vi "Main Loop.vi"(8 "error in":errorcluster, 11 "Node in":refnum<class "BLS Chiller Template.lvclass">) -> (0 "error out":errorcluster, 3 "Node out":refnum<class "BLS Chiller Template.lvclass">)   [LabVIEW 2023, in "BLS Chiller Template.lvlib" / "BLS Chiller Template.lvclass"]
uses:
  BLS Chiller Template.lvclass
  Out Of Band/Type Defs/gRPC to Main.ctl
  Out Of Band/Type Defs/Main to gRPC.ctl
  <vilib>/ADAS Replay HIL/ADAS Plugin Utilities/AdasLvTemplate/Typedefs/Initialization States.ctl
  <vilib>/ADAS Replay HIL/ADAS Plugin Utilities/AdasLvTemplate/AdasLvTemplate.lvclass/AdasLvTemplate.ctl
  <vilib>/Platform/TimedLoop/XDataNode/timing_clust.ctl
  <vilib>/Platform/TimedLoop/XDataNode/nitl_modes.ctl
  <vilib>/Platform/TimedLoop/XDataNode/wakeup.ctl
  <vilib>/ADAS Replay HIL/ADAS Plugin Utilities/AdasLvTemplate/Typedefs/Default Plug-in States.ctl
  <vilib>/ADAS Replay HIL/ADAS Plugin Utilities/AdasLvTemplateTimeLog/Typedefs/Standard Time Events.ctl
  <vilib>/ADAS Replay HIL/ADAS Plugin Utilities/AdasLvTemplate/Typedefs/Error Options.ctl
  <vilib>/ADAS Replay HIL/Template Node/Plugin/Template Node/Template Node.lvclass/Template Node.ctl
  <vilib>/ADAS Replay HIL/ADAS Plugin Utilities/AdasLvTemplate/Time/Absolute Timed Wake.vi
  <vilib>/ADAS Replay HIL/ADAS Plugin Utilities/AdasLvTemplate/OOB Commands/OOB Comm.vi
  <vilib>/ADAS Replay HIL/ADAS Plugin Utilities/AdasLvTemplate/Time/Get Current Working Time.vi
  <vilib>/ADAS Replay HIL/ADAS Plugin Utilities/AdasLvTemplate/Time/Wake on Time.vi
  <vilib>/ADAS Replay HIL/ADAS Plugin Utilities/AdasLvTemplate/TimeLog/Write Timelog.vi
  Out Of Band/Main Loop/Main OOB Comm.vi
  Out Of Band/gRPC Loop/gRPC OOB Comm.vi
  <vilib>/ADAS Replay HIL/ADAS Plugin Utilities/AdasLvTemplate/Time/Sleep on Working Time.vi
  <vilib>/ADAS Replay HIL/ADAS Plugin Utilities/AdasLvTemplateSystemLog/Syslog Info.vi
  <vilib>/ADAS Replay HIL/ADAS Plugin Utilities/AdasLvTemplate/OOB Commands/Parse Timing Data.vi
  <vilib>/ADAS Replay HIL/ADAS Plugin Utilities/AdasLvTemplate/OOB Commands/Typecast Command ID.vi
  <vilib>/ADAS Replay HIL/ADAS Plugin Utilities/AdasLvTemplate/OOB Responses/Write Status.vi
  <vilib>/ADAS Replay HIL/ADAS Plugin Utilities/AdasLvTemplateOutOfBand/Read OOB no_mem.vi
  <vilib>/ADAS Replay HIL/ADAS Plugin Utilities/AdasLvTemplateCommon/Time/Calculate Cycle Timing Statistics.vi
  <vilib>/ADAS Replay HIL/ADAS Plugin Utilities/AdasLvTemplateCommon/Time/Calculate Delta Timing Statistics.vi
  <vilib>/ADAS Replay HIL/ADAS Plugin Utilities/AdasLvTemplate/OOB Responses/Update StatusPub Timing Stats.vi
  <vilib>/ADAS Replay HIL/ADAS Plugin Utilities/AdasLvTemplate/TimeLog/Write All States Timelog.vi
  <vilib>/ADAS Replay HIL/ADAS Plugin Utilities/AdasLvTemplate/TimeLog/Update Data Output Timing Stats.vi
  <vilib>/ADAS Replay HIL/ADAS Plugin Utilities/AdasLvTemplateSystemLog/Write to ADAS Log.vi
  <vilib>/ADAS Replay HIL/ADAS Plugin Utilities/AdasLvTemplateCommon/Byte Pack/Unpack Data.vi
  <vilib>/ADAS Replay HIL/ADAS Plugin Utilities/AdasLvTemplateCommon/Byte Pack/Unpack U64.vi
  <vilib>/ADAS Replay HIL/ADAS Plugin Utilities/AdasLvTemplateCommon/Byte Pack/Unpack Dbl.vi
  <vilib>/ADAS Replay HIL/ADAS Plugin Utilities/AdasLvTemplate/OOB Commands/Typecast Command ID.vi/33a1a329-153d-46bf-b82a-13d67c924fdc.vi
  <vilib>/ADAS Replay HIL/ADAS Plugin Utilities/AdasLvTemplate/OOB Commands/Typecast Command ID.vi/47c6e19f-85af-4ecd-9b35-4c0af7f9c4eb.vi
  <vilib>/ADAS Replay HIL/ADAS Plugin Utilities/AdasLvTemplate/OOB Responses/Send Status.vi
  <vilib>/ADAS Replay HIL/ADAS Plugin Utilities/AdasLvTemplateCommon/Byte Pack/Unpack U8.vi
  <vilib>/ADAS Replay HIL/ADAS Plugin Utilities/AdasLvTemplateTimeLog/Write All State Timelog.vi
  <vilib>/ADAS Replay HIL/ADAS Plugin Utilities/AdasLvTemplate/TimeLog/Write All Data Outputs Timelog.vi
  <vilib>/ADAS Replay HIL/ADAS Plugin Utilities/AdasLvTemplateSystemLog/Log to OS.vi
  <vilib>/ADAS Replay HIL/ADAS Plugin Utilities/AdasLvTemplateCommon/Byte Pack/Unpack U64.vi/6cead1c8-1490-489b-94c0-a6f77a877bd8.vi
  <vilib>/ADAS Replay HIL/ADAS Plugin Utilities/AdasLvTemplateCommon/Byte Pack/Unpack Dbl.vi/1ddba392-4989-4550-9efa-bf0f5b4d8642.vi
  <vilib>/ADAS Replay HIL/ADAS Plugin Utilities/AdasLvTemplate/OOB Commands/Typecast Command ID.vi/33a1a329-153d-46bf-b82a-13d67c924fdc.vi/c28b0ead-42ad-4072-80a2-aca7f2bd7ce3.vi
  <vilib>/ADAS Replay HIL/ADAS Plugin Utilities/AdasLvTemplate/OOB Commands/Typecast Command ID.vi/47c6e19f-85af-4ecd-9b35-4c0af7f9c4eb.vi/c28b0ead-42ad-4072-80a2-aca7f2bd7ce3.vi
  <vilib>/ADAS Replay HIL/ADAS Plugin Utilities/AdasLvTemplate/OOB Responses/Pack Status.vi
  <vilib>/ADAS Replay HIL/ADAS Plugin Utilities/AdasLvTemplateOutOfBand/Write OOB no_mem.vi
  <vilib>/ADAS Replay HIL/ADAS Plugin Utilities/AdasLvTemplateCommon/Byte Pack/Unpack U8.vi/dab2b46f-2b54-43c4-abff-a01388689065.vi
  <vilib>/ADAS Replay HIL/ADAS Plugin Utilities/AdasLvTemplateTimeLog/Write Standard Timelog.vi
  <vilib>/ADAS Replay HIL/ADAS Plugin Utilities/AdasLvTemplateTimeLog/Write Data Channel Timelog.vi
  <vilib>/ADAS Replay HIL/ADAS Plugin Utilities/AdasLvTemplateCommon/Byte Pack/Unpack U64.vi/6cead1c8-1490-489b-94c0-a6f77a877bd8.vi/c28b0ead-42ad-4072-80a2-aca7f2bd7ce3.vi
  <vilib>/ADAS Replay HIL/ADAS Plugin Utilities/AdasLvTemplateCommon/Byte Pack/Unpack Dbl.vi/1ddba392-4989-4550-9efa-bf0f5b4d8642.vi/c28b0ead-42ad-4072-80a2-aca7f2bd7ce3.vi
  <vilib>/ADAS Replay HIL/ADAS Plugin Utilities/AdasLvTemplate/OOB Responses/Pack Status.vi/b11e0591-7eee-4cf7-b3b4-c7ab44274ca8.vi
  <vilib>/ADAS Replay HIL/ADAS Plugin Utilities/AdasLvTemplateCommon/Byte Pack/Pack Data.vi
  <vilib>/ADAS Replay HIL/ADAS Plugin Utilities/AdasLvTemplateCommon/Byte Pack/Pack U8.vi
  <vilib>/ADAS Replay HIL/ADAS Plugin Utilities/AdasLvTemplateCommon/Byte Pack/Unpack U8.vi/dab2b46f-2b54-43c4-abff-a01388689065.vi/c28b0ead-42ad-4072-80a2-aca7f2bd7ce3.vi
  <vilib>/ADAS Replay HIL/ADAS Plugin Utilities/AdasLvTemplateTimeLog/Write Standard Timelog.vi/f085caac-7a92-4bf8-966d-28d65be49b40.vi
  <vilib>/ADAS Replay HIL/ADAS Plugin Utilities/AdasLvTemplate/Time/Get Current System Time.vi
  <vilib>/ADAS Replay HIL/ADAS Plugin Utilities/AdasLvTemplateSystemLog/Syslog to bytes.vi
  <vilib>/ADAS Replay HIL/ADAS Plugin Utilities/AdasLvTemplate/OOB Responses/Pack Status.vi/b11e0591-7eee-4cf7-b3b4-c7ab44274ca8.vi/c28b0ead-42ad-4072-80a2-aca7f2bd7ce3.vi
  <vilib>/ADAS Replay HIL/ADAS Plugin Utilities/AdasLvTemplateCommon/Byte Pack/Pack U8.vi/d26b960e-7005-4648-98c8-b1ee87e9a649.vi
  <vilib>/libnicipc/SubVIs/check_error.vi
  <vilib>/libnicipc/Get Element Write Position.vi
  <vilib>/ADAS Replay HIL/ADAS Plugin Utilities/AdasLvTemplateCommon/Byte Pack/Pack U16.vi
  <vilib>/ADAS Replay HIL/ADAS Plugin Utilities/AdasLvTemplateCommon/Byte Pack/Pack U64.vi
  <vilib>/ADAS Replay HIL/ADAS Plugin Utilities/AdasLvTemplateCommon/Byte Pack/Pack U8.vi/d26b960e-7005-4648-98c8-b1ee87e9a649.vi/c28b0ead-42ad-4072-80a2-aca7f2bd7ce3.vi
  <vilib>/ADAS Replay HIL/ADAS Plugin Utilities/AdasLvTemplateCommon/Byte Pack/Pack U16.vi/b7087905-2eb2-4c97-90c8-7b5681595cff.vi
  <vilib>/ADAS Replay HIL/ADAS Plugin Utilities/AdasLvTemplateCommon/Byte Pack/Pack U64.vi/5a0cf944-c84d-49bc-a60a-1e686f5e9f60.vi
  <vilib>/ADAS Replay HIL/ADAS Plugin Utilities/AdasLvTemplateCommon/Byte Pack/Pack U16.vi/b7087905-2eb2-4c97-90c8-7b5681595cff.vi/c28b0ead-42ad-4072-80a2-aca7f2bd7ce3.vi
  <vilib>/ADAS Replay HIL/ADAS Plugin Utilities/AdasLvTemplateCommon/Byte Pack/Pack U64.vi/5a0cf944-c84d-49bc-a60a-1e686f5e9f60.vi/c28b0ead-42ad-4072-80a2-aca7f2bd7ce3.vi
  Out Of Band/gRPC Loop/Class to gRPC_to_Main.vi
  Out Of Band/Main Loop/Class to Main_to_gRPC.vi
  <vilib>/ADAS Replay HIL/ADAS Plugin Utilities/AdasLvTemplate/OOB Commands/Parse Start Restart Data.vi
  <vilib>/ADAS Replay HIL/ADAS Plugin Utilities/AdasLvTemplate/OOB Commands/Parse Priority Data.vi
  <vilib>/ADAS Replay HIL/AdasHilServices/Get Time.vi
  <vilib>/ADAS Replay HIL/AdasHilServices/nS Sleep.vi
  <vilib>/Utility/error.llb/Error Cluster From Error Code.vi
  <vilib>/ADAS Replay HIL/AdasHilServices/Wake On Time Advanced.vi
  <vilib>/libnicipc/SubVIs/Get Element Info Variant.vi
  <vilib>/libnicipc/Notify Of New Write.vi
  <vilib>/ADAS Replay HIL/ADAS Plugin Utilities/AdasLvTemplate/AdasLvTemplate.lvclass
  <vilib>/Platform/TimedLoop/XDataNode/XDataNode.xnode
  BLS Chiller Template.lvclass/BLS Chiller Template.ctl
  <vilib>/ADAS Replay HIL/Template Node/Plugin/Template Node/Template Node.lvclass
  <vilib>/ADAS Replay HIL/ADAS Plugin Utilities/AdasLvTemplateTimeLog/AdasLvTemplateTimeLog.lvlib
  <vilib>/Platform/TimedLoop/XDataNode/XDNodeRunTimeDep.lvlib
panel:
  out "Main to gRPC":T1
  out "gRPC to Main":T2
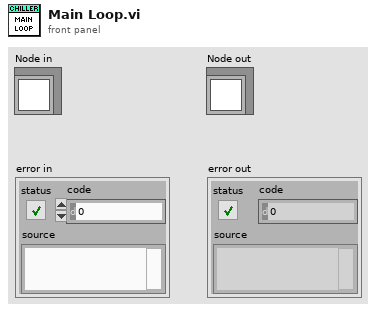
[diagram p1: front panel]
types:
  T1 = typedef "BLS Chiller Template.lvlib/BLS Chiller Template.lvclass/Main to gRPC.ctl" = cluster{"void":bool}
  T2 = typedef "BLS Chiller Template.lvlib/BLS Chiller Template.lvclass/gRPC to Main.ctl" = cluster{"void":bool}
  T3 = typedef "AdasLvTemplate.lvlib/AdasLvTemplate.lvclass/Initialization States.ctl" = enum16{"Entry Init", "Ready", "Exit Init", "Error"}
  T4 = typedef "AdasLvTemplate.lvlib/AdasLvTemplate.lvclass/Default Plug-in States.ctl" = enum16{"Start", "Pause", "Restart", "Execute Logic", "Housekeeping", "Error", "Shutdown"}
  T5 = typedef "AdasLvTemplateTimeLog.lvlib/Standard Time Events.ctl" = enum16{"Start Sleep", "Wakeup", "End of Execution", "Start of Housekeeping", "Target Wake Time", "Channel T0", "Channel TX_in", "Channel RX", "Channel out", "Target Channel out "}
  T6 = typedef "AdasLvTemplate.lvlib/AdasLvTemplate.lvclass/Error Options.ctl" = enum16{"Clear and Log Only", "Pause on Error", "Restart on Error", "Pause on Warning", "Restart on Warning"}
  T7 = typedef "XDNodeRunTimeDep.lvlib/timing_clust.ctl" = cluster{"Expected End [f-1]":u64, "Actual End [f-1]":u64, "Finished Late? [f-1]":bool, "Expected End [i-1]":u64, "Actual End [i-1]":u64, "Finished Late? [i-1]":bool, "Expected Start [i]":u64, "Actual Start [i]":u64, "Expected Start [f]":u64, "Actual Start [f]":u64, "Source Name":string, "Structure Name":string, "Period":i64, "Deadline":i64, "Offset":i64, "Start":i64, "Priority":i32, "Timeout":i32, "Mode":T8, "Wakeup Reason":T9, "Error":errorcluster, "Source Type":string, "Secondary Source Type":string, "Global End Time":u64, "Global Start Time":u64, "Frame Duration":u64, "Iteration Duration":u64, "Assigned CPU":i32, "I/O Scan Engine Mode":u32}
  T8 = typedef "XDNodeRunTimeDep.lvlib/nitl_modes.ctl" = enum32{"No Change", "Process missed periods, maintain original phase", "Discard missed periods, maintain original phase", "Process missed periods, ignore original phase", "Discard missed periods, ignore original phase"}
  T9 = typedef "XDNodeRunTimeDep.lvlib/wakeup.ctl" = enum32{"Normal", "Aborted", "Asynchronous wakeup", "Timing source error", "Timed loop error", "Timeout"}
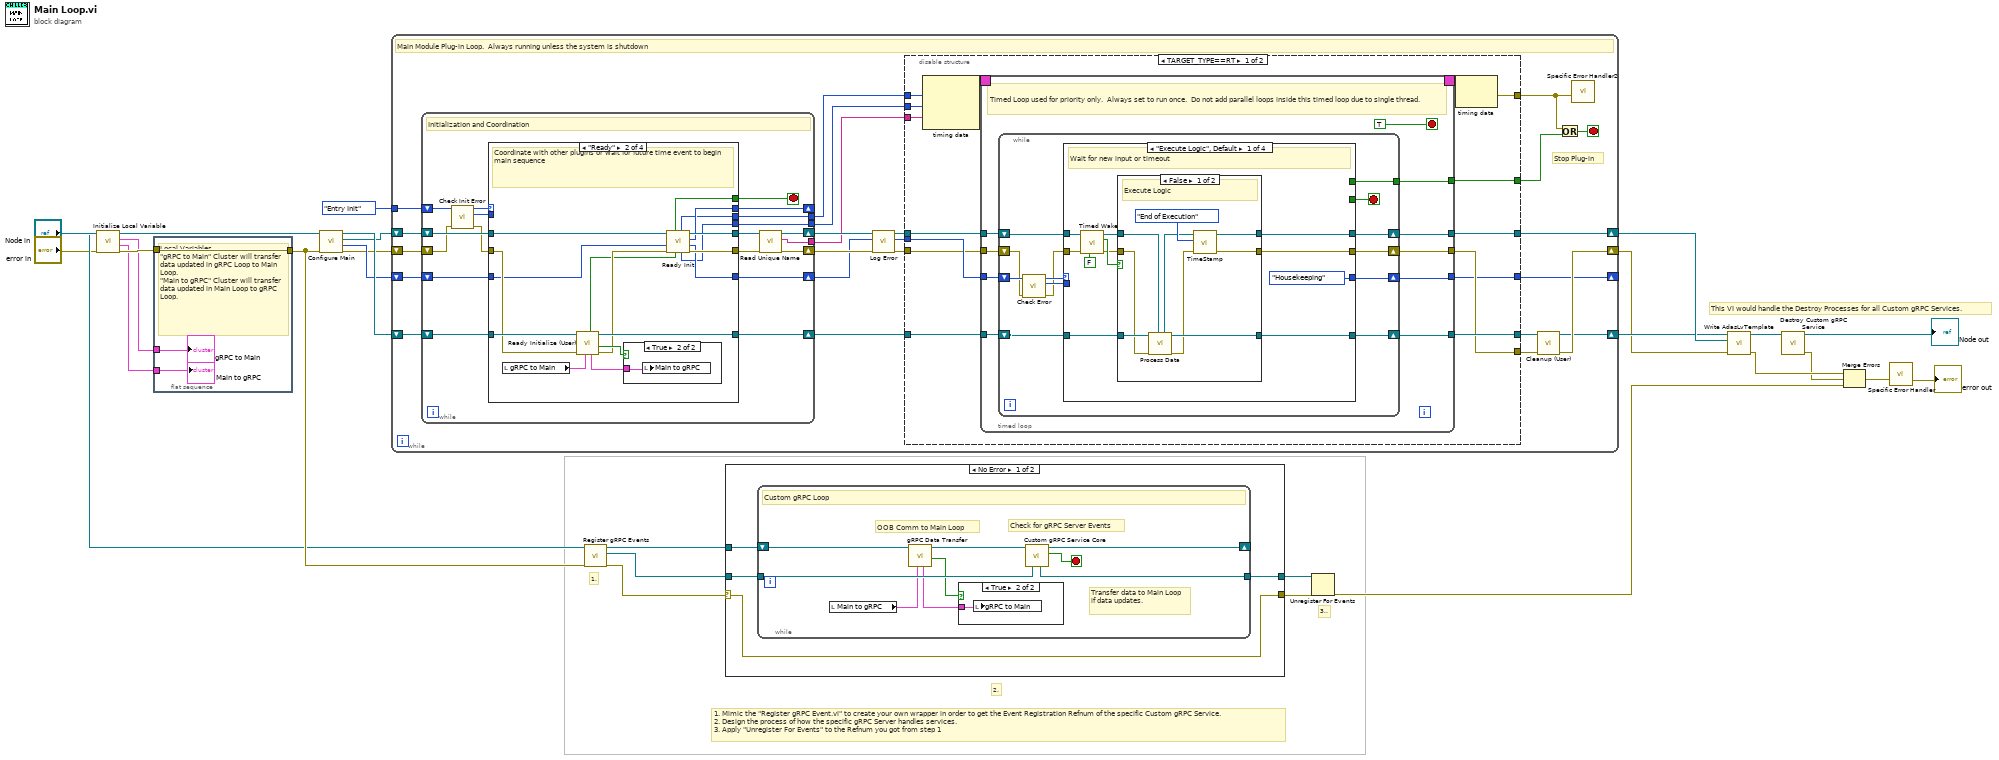
[diagram p0: block diagram]
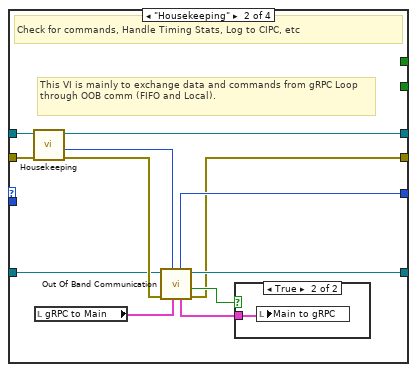
[diagram p5: hidden frame]
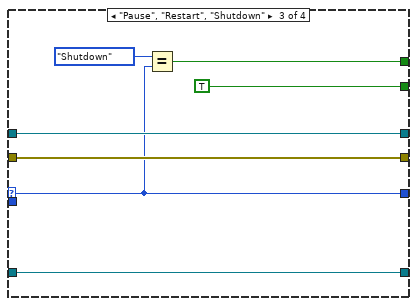
[diagram p7: hidden frame]
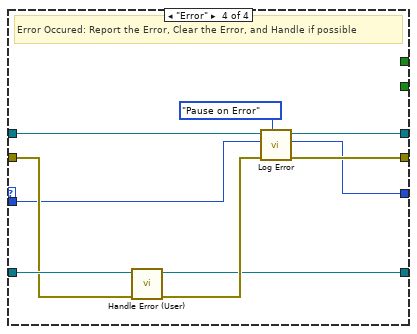
[diagram p8: hidden frame]
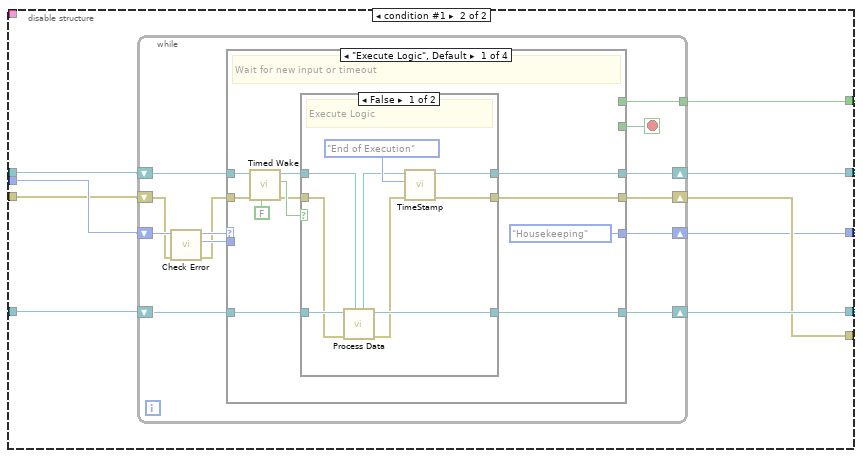
[diagram p9: hidden frame]
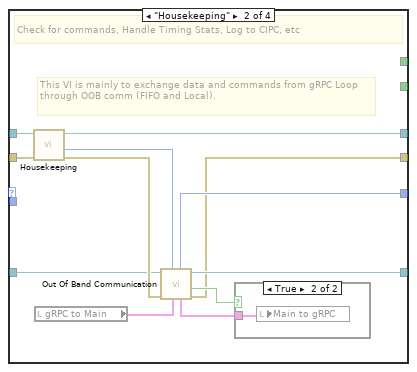
[diagram p11: hidden frame]
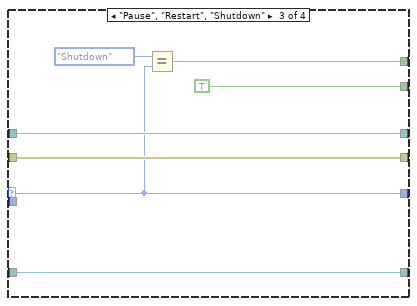
[diagram p13: hidden frame]
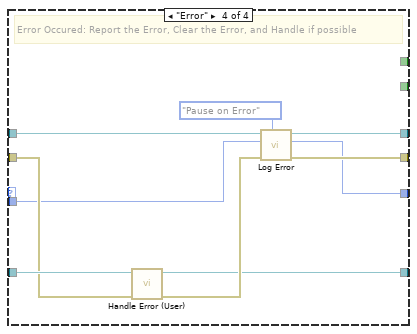
[diagram p14: hidden frame]
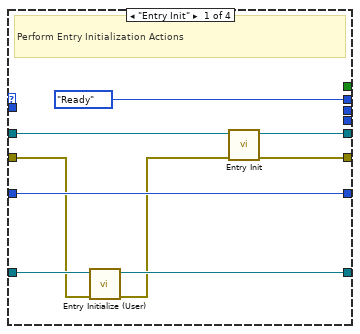
[diagram p15: hidden frame]
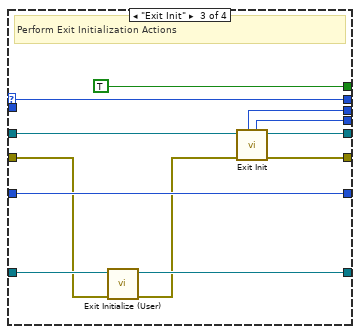
[diagram p17: hidden frame]
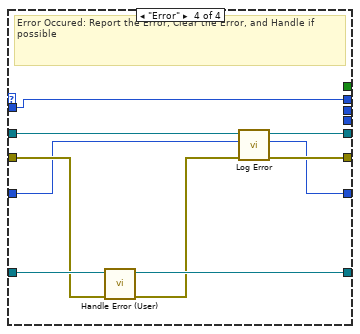
[diagram p18: hidden frame]
diagram:
  # "This VI would handle the Destroy Processes for all Custom gRPC Services."
  # "3.."
  # "2."
  # "1."
  # "1. Mimic the \"Register gRPC Event.vi\" to create your own wrapper in order to get the Event Registration Refnum of the specific Custom gRPC Service.\n2. Design the process of how the specific gRPC Server handles services.\n3. Apply \"Unregister For Events\" to the Refnum you got from step 1"
  n1 = call "Initialize Local Variable.vi"("error in"="error in", "Timed Node in"="Node in") -> ("error out"=w5:errorcluster, "Main to gRPC"=w3:T1, "gRPC to Main"=w4:T2, "Timed Node out"=w7:refnum<class "BLS Chiller Template.lvclass">)  [unwired: 6 in]
  n2 = flat-sequence {
    tunnel: w5 -> [w30]
    tunnel: [w30] -> w9
    tunnel: w4 -> [w29]
    tunnel: w3 -> [w28]
    frame #0 {
      # "Local Variables \n\"gRPC to Main\" Cluster will transfer data updated in gRPC Loop to Main Loop.\n\"Main to gRPC\" Cluster will transfer data updated in Main Loop to gRPC Loop."
      "gRPC to Main" <- w29
      "Main to gRPC" <- w28
    }
  }
  n3 = call <vilib>:"Configure Main.vi"("error in (no error)"=w9, "Template Node in"=w7) -> ("error out"=w21:errorcluster, "Initial State"=w22:T4, "AdasLvTemplate"=w20:refnum<class "AdasLvTemplate.lvclass">, "Template Node out"=w23:refnum<class "BLS Chiller Template.lvclass">)  [unwired: 6 in]
  n4 = while {
    shift-right: [w38] -> w27
    shift-left: w20 -> [w51]
    shift-right: [w36] -> _
    shift-left: w22 -> [w53]
    shift-right: [w46] -> w26
    shift-left: w23 -> [w54]
    shift-right: [w47] -> w25
    shift-left: w21 -> [w52]
    tunnel: Initialization_States."Entry Init" -> [w50]
    stop <- w45 stop-if-true
    # "Stop Plug-in"
    # "Main Module Plug-in Loop.  Always running unless the system is shutdown"
    n5 = while {
      shift-right: [w248] -> _
      shift-left: w50 -> [w242]
      shift-right: [w231] -> w49
      shift-left: w51 -> [w246]
      shift-right: [w233] -> w48
      shift-left: w52 -> [w240]
      shift-right: [w243] -> w43
      shift-left: w54 -> [w244]
      shift-right: [w237] -> w44
      shift-left: w53 -> [w236]
      tunnel: [w235] -> w31
      tunnel: [w234] -> w32
      tunnel: [w230] -> w33
      stop <- w247 stop-if-true
      # "Initialization and Coordination"
      n6 = call <vilib>:"Check Init Error.vi"("error in"=w240, "State"=w242) -> ("error out"=w239:errorcluster, "Next State"=w238:T3, "State"=w241:T3)  [unwired: 7 in]
      n7 = case shown="\"Ready\"" w241 {
        selector: w241 -> [_ _ w287 _]
        tunnel: [Initialization_States."Ready" w264 w287 w295] -> w248
        tunnel: [_ w259 TRUE ("stop 2") _] -> w247
        tunnel: w246 -> [w250 w274 w276 w290]
        tunnel: [w255 w273 w283 w297] -> w232
        tunnel: [w249 w267 w282 w296] -> w245
        tunnel: w238 -> [_ _ _ w295]
        tunnel: w239 -> [w251 w265 w277 w291]
        tunnel: w244 -> [w254 w272 w280 w294]
        tunnel: [w253 w271 w279 w293] -> w243
        tunnel: [w256 w262 w281 w289] -> w237
        tunnel: w236 -> [w256 w261 w281 w288]
        tunnel: [_ w263 w285 _] -> w235
        tunnel: [_ w260 w284 _] -> w234
        frame "Entry Init" {
          # "Perform Entry Initialization Actions"
          n8 = call "Entry Initialize (User).vi"("error in"=w251, "Node in"=w254) -> ("error out"=w252:errorcluster, "Node out"=w253:refnum<class "BLS Chiller Template.lvclass">)  [unwired: 8 in]
          n9 = call <vilib>:"Entry Init.vi"("error in (no error)"=w252, "AdasLvTemplate in"=w250) -> ("error out"=w249:errorcluster, "AdasLvTemplate out"=w255:refnum<class "AdasLvTemplate.lvclass">)  [unwired: 8 in]
        }
        frame "Ready" {
          # "Coordinate with other plugins or wait for future time event to begin main sequence"
          n10 = local read "gRPC to Main"() -> (w269:T2)
          n11 = call "Ready Initialize (User).vi"("gRPC to Main"=w269, "error in (no error)"=w265, "Node in"=w272) -> ("error out"=w266:errorcluster, "Update Local Variable"=w270:bool, "Node out"=w271:refnum<class "BLS Chiller Template.lvclass">, "Main to gRPC"=w268:T1, "User Ready Init Done"=w258:bool)  [unwired: 4 in]
          n12 = case shown="True" w270 {
            tunnel: w268 -> [_ w275]
            frame False {
            }
            frame True {
              n13 = local write "Main to gRPC"(w275) -> ()
            }
          }
          n14 = call <vilib>:"Ready Init.vi"("User Ready Init Done"=w258, "error in (no error)"=w266, "Plug-in State in"=w261, "AdasLvTemplate in"=w274) -> ("error out"=w267:errorcluster, "Plug-in State"=w262:T4, "Initialization State"=w264:T3, "AdasLvTemplate out"=w273:refnum<class "AdasLvTemplate.lvclass">, "Processor"=w260:i32, "Priority"=w263:i32, "Shutdown?"=w259:bool)  [unwired: 1 in]
        }
        frame "Exit Init" {
          # "Perform Exit Initialization Actions"
          n15 = call "Exit Initialize (User).vi"("error in"=w277, "Node in"=w280) -> ("error out"=w278:errorcluster, "Node out"=w279:refnum<class "BLS Chiller Template.lvclass">)  [unwired: 8 in]
          n16 = call <vilib>:"Exit Init.vi"("error in (no error)"=w278, "AdasLvTemplate in"=w276) -> ("error out"=w282:errorcluster, "AdasLvTemplate out"=w283:refnum<class "AdasLvTemplate.lvclass">, "Processor"=w284:i32, "Priority"=w285:i32)  [unwired: 5 in, 1 out]
        }
        frame "Error" {
          # "Error Occured: Report the Error, Clear the Error, and Handle if possible"
          n17 = call "Handle Error (User).vi"("error in"=w291, "Node in"=w294) -> ("error out"=w292:errorcluster, "Node out"=w293:refnum<class "BLS Chiller Template.lvclass">)  [unwired: 8 in]
          n18 = call <vilib>:"Log Error.vi"("error in (no error)"=w292, "Plug-in State in"=w288, "AdasLvTemplate in"=w290) -> ("error out"=w296:errorcluster, "Plug-in State out"=w289:T4, "AdasLvTemplate out"=w297:refnum<class "AdasLvTemplate.lvclass">)  [unwired: 6 in]
        }
      }
      n19 = call <vilib>:"Read Unique Name.vi"("error in"=w245, "AdasLvTemplate in"=w232) -> ("error out"=w233:errorcluster, "Unique Name"=w230:string, "AdasLvTemplate out"=w231:refnum<class "AdasLvTemplate.lvclass">)  [unwired: 7 in]
    }
    n20 = call <vilib>:"Log Error.vi"("error in (no error)"=w48, "Plug-in State in"=w44, "AdasLvTemplate in"=w49) -> ("error out"=w40:errorcluster, "Plug-in State out"=w41:T4, "AdasLvTemplate out"=w39:refnum<class "AdasLvTemplate.lvclass">)  [unwired: 6 in]
    n21 = disable-structure shown="TARGET_TYPE==RT" {
      disable-tunnel: w43 -> [w67 w163]
      disable-tunnel: [w66 w162] -> w42
      disable-tunnel: w41 -> [w65 w161]
      disable-tunnel: w40 -> [w64 w160]
      disable-tunnel: w39 -> [w63 w159]
      disable-tunnel: [w62 w158] -> w38
      disable-tunnel: [w61 w157] -> w37
      disable-tunnel: [w60 w156] -> w36
      disable-tunnel: [w59 w155] -> w35
      disable-tunnel: [w58 _] -> w34
      disable-tunnel: w33 -> [w57 _]
      disable-tunnel: w32 -> [w56 _]
      disable-tunnel: w31 -> [w55 _]
      frame condition #0 (active) {
        n22 = node-c288(w55, w56, w57) -> (w69:T7)
        n23 = timed-loop {
          timing: w69 -> [_]
          timing-out: [_] -> w68
          tunnel: w67 -> [w79]
          tunnel: [w78] -> w66
          tunnel: w65 -> [w77]
          tunnel: w64 -> [w76]
          tunnel: w63 -> [w75]
          tunnel: [w74] -> w62
          tunnel: [w73] -> w61
          tunnel: [w72] -> w60
          tunnel: [w71] -> w59
          stop <- TRUE stop-if-true
          # "Timed Loop used for priority only.  Always set to run once.  Do not add parallel loops inside this timed loop due to single thread."
          n24 = while {
            shift-right: [w92] -> w72
            shift-left: w77 -> [w86]
            tunnel: [w90] -> w71
            shift-right: [w88] -> w74
            shift-left: w75 -> [w89]
            shift-right: [w87] -> w73
            shift-left: w76 -> [w83]
            shift-right: [w81] -> w78
            shift-left: w79 -> [w82]
            stop <- w91 stop-if-true
            n25 = call <vilib>:"Check Error.vi"("error in"=w83, "State"=w86) -> ("error out"=w80:errorcluster, "Next State"=w84:T4, "State"=w85:T4)  [unwired: 7 in]
            n26 = case shown="\"Execute Logic\", Default" w85 {
              selector: w85 -> [_ _ w130 _]
              tunnel: [Default_Plug-in_States."Housekeeping" ("Default Plug-in States") w123 w130 w138] -> w92
              tunnel: [_ _ TRUE ("stop 2") _] -> w91
              tunnel: [_ _ w129 _] -> w90
              tunnel: w89 -> [w97 w127 w135 w139]
              tunnel: [w99 w125 w135 w145] -> w88
              tunnel: [w93 w116 w133 w144] -> w87
              tunnel: w84 -> [_ _ _ w136]
              tunnel: w80 -> [w98 w126 w133 w142]
              tunnel: w82 -> [w96 w121 w132 w143]
              tunnel: [w95 w120 w132 w140] -> w81
              frame "Execute Logic", Default {
                # "Wait for new input or timeout"
                n27 = call <vilib>:"Timed Wake.vi"("Data Driven Timing"=FALSE, "error in (no error)"=w98, "AdasLvTemplate in"=w97) -> ("error out"=w100:errorcluster, "Timeout"=w103:bool, "AdasLvTemplate out"=w101:refnum<class "AdasLvTemplate.lvclass">)  [unwired: 4 in, 2 out]
                n28 = case shown="False" w103 {
                  tunnel: [w108 w115] -> w99
                  tunnel: w101 -> [w106 w115]
                  tunnel: [w104 w114] -> w93
                  tunnel: w100 -> [w109 w114]
                  tunnel: w96 -> [w111 w113]
                  tunnel: [w110 w113] -> w95
                  frame False {
                    # "Execute Logic"
                    n29 = call "Process Data.vi"("AdasLvTemplate in"=w106, "error in"=w109, "Node in"=w111) -> ("error out"=w107:errorcluster, "Node out"=w110:refnum<class "BLS Chiller Template.lvclass">, "AdasLvTemplate out"=w105:refnum<class "AdasLvTemplate.lvclass">)  [unwired: 6 in]
                    n30 = call <vilib>:"TimeStamp.vi"("error in (no error)"=w107, "Event"=Standard_Time_Events."End of Execution", "AdasLvTemplate in"=w105) -> ("error out"=w104:errorcluster, "AdasLvTemplate out"=w108:refnum<class "AdasLvTemplate.lvclass">)  [unwired: 7 in]
                  }
                  frame True {
                    # "Timeout"
                  }
                }
              }
              frame "Housekeeping" {
                # "This VI is mainly to exchange data and commands from gRPC Loop through OOB comm (FIFO and Local)."
                # "Check for commands, Handle Timing Stats, Log to CIPC, etc"
                n31 = call <vilib>:"Housekeeping.vi"("error in (no error)"=w126, "AdasLvTemplate in"=w127) -> ("error out"=w122:errorcluster, "State"=w124:T4, "AdasLvTemplate out"=w125:refnum<class "AdasLvTemplate.lvclass">)  [unwired: 7 in]
                n32 = local read "gRPC to Main"() -> (w119:T2)
                n33 = call "Out Of Band Communication.vi"("gRPC to Main"=w119, "State In"=w124, "error in"=w122, "Node in"=w121) -> ("error out"=w116:errorcluster, "Update Local Variable"=w117:bool, "Node out"=w120:refnum<class "BLS Chiller Template.lvclass">, "Main to gRPC"=w118:T1, "State Out"=w123:T4)  [unwired: 3 in]
                n34 = case shown="True" w117 {
                  tunnel: w118 -> [_ w128]
                  frame False {
                  }
                  frame True {
                    n35 = local write "Main to gRPC"(w128) -> ()
                  }
                }
              }
              frame "Pause", "Restart", "Shutdown" {
                n36 = Equal?(x=Default_Plug-in_States."Shutdown" ("Default Plug-in States"), y=w130) -> (x = y?=w129:bool)
              }
              frame "Error" {
                # "Error Occured: Report the Error, Clear the Error, and Handle if possible"
                n37 = call "Handle Error (User).vi"("error in"=w142, "Node in"=w143) -> ("error out"=w141:errorcluster, "Node out"=w140:refnum<class "BLS Chiller Template.lvclass">)  [unwired: 8 in]
                n38 = call <vilib>:"Log Error.vi"("Action"=Error_Options."Pause on Error", "error in (no error)"=w141, "Plug-in State in"=w136, "AdasLvTemplate in"=w139) -> ("error out"=w144:errorcluster, "Plug-in State out"=w138:T4, "AdasLvTemplate out"=w145:refnum<class "AdasLvTemplate.lvclass">)  [unwired: 5 in]
              }
            }
          }
        }
        n39 = node-c288(w68) -> (w58:errorcluster)
      }
      frame condition #1 {
        n40 = while {
          shift-right: [w176] -> w156
          shift-left: w161 -> [w170]
          tunnel: [w174] -> w155
          shift-right: [w172] -> w158
          shift-left: w159 -> [w173]
          shift-right: [w171] -> w157
          shift-left: w160 -> [w167]
          shift-right: [w165] -> w162
          shift-left: w163 -> [w166]
          stop <- w175 stop-if-true
          n41 = call <vilib>:"Check Error.vi"("error in"=w167, "State"=w170) -> ("error out"=w164:errorcluster, "Next State"=w168:T4, "State"=w169:T4)  [unwired: 7 in]
          n42 = case shown="\"Execute Logic\", Default" w169 {
            selector: w169 -> [_ _ w214 _]
            tunnel: [Default_Plug-in_States."Housekeeping" ("Default Plug-in States") w207 w214 w222] -> w176
            tunnel: [_ _ TRUE ("stop 2") _] -> w175
            tunnel: [_ _ w213 _] -> w174
            tunnel: w173 -> [w181 w211 w219 w223]
            tunnel: [w183 w209 w219 w229] -> w172
            tunnel: [w177 w200 w217 w228] -> w171
            tunnel: w168 -> [_ _ _ w220]
            tunnel: w164 -> [w182 w210 w217 w226]
            tunnel: w166 -> [w180 w205 w216 w227]
            tunnel: [w179 w204 w216 w224] -> w165
            frame "Execute Logic", Default {
              # "Wait for new input or timeout"
              n43 = call <vilib>:"Timed Wake.vi"("Data Driven Timing"=FALSE, "error in (no error)"=w182, "AdasLvTemplate in"=w181) -> ("error out"=w184:errorcluster, "Timeout"=w187:bool, "AdasLvTemplate out"=w185:refnum<class "AdasLvTemplate.lvclass">)  [unwired: 4 in, 2 out]
              n44 = case shown="False" w187 {
                tunnel: [w192 w199] -> w183
                tunnel: w185 -> [w190 w199]
                tunnel: [w188 w198] -> w177
                tunnel: w184 -> [w193 w198]
                tunnel: w180 -> [w195 w197]
                tunnel: [w194 w197] -> w179
                frame False {
                  # "Execute Logic"
                  n45 = call "Process Data.vi"("AdasLvTemplate in"=w190, "error in"=w193, "Node in"=w195) -> ("error out"=w191:errorcluster, "Node out"=w194:refnum<class "BLS Chiller Template.lvclass">, "AdasLvTemplate out"=w189:refnum<class "AdasLvTemplate.lvclass">)  [unwired: 6 in]
                  n46 = call <vilib>:"TimeStamp.vi"("error in (no error)"=w191, "Event"=Standard_Time_Events."End of Execution", "AdasLvTemplate in"=w189) -> ("error out"=w188:errorcluster, "AdasLvTemplate out"=w192:refnum<class "AdasLvTemplate.lvclass">)  [unwired: 7 in]
                }
                frame True {
                  # "Timeout"
                }
              }
            }
            frame "Housekeeping" {
              # "This VI is mainly to exchange data and commands from gRPC Loop through OOB comm (FIFO and Local)."
              # "Check for commands, Handle Timing Stats, Log to CIPC, etc"
              n47 = call <vilib>:"Housekeeping.vi"("error in (no error)"=w210, "AdasLvTemplate in"=w211) -> ("error out"=w206:errorcluster, "State"=w208:T4, "AdasLvTemplate out"=w209:refnum<class "AdasLvTemplate.lvclass">)  [unwired: 7 in]
              n48 = local read "gRPC to Main"() -> (w203:T2)
              n49 = call "Out Of Band Communication.vi"("gRPC to Main"=w203, "State In"=w208, "error in"=w206, "Node in"=w205) -> ("error out"=w200:errorcluster, "Update Local Variable"=w201:bool, "Node out"=w204:refnum<class "BLS Chiller Template.lvclass">, "Main to gRPC"=w202:T1, "State Out"=w207:T4)  [unwired: 3 in]
              n50 = case shown="True" w201 {
                tunnel: w202 -> [_ w212]
                frame False {
                }
                frame True {
                  n51 = local write "Main to gRPC"(w212) -> ()
                }
              }
            }
            frame "Pause", "Restart", "Shutdown" {
              n52 = Equal?(x=Default_Plug-in_States."Shutdown" ("Default Plug-in States"), y=w214) -> (x = y?=w213:bool)
            }
            frame "Error" {
              # "Error Occured: Report the Error, Clear the Error, and Handle if possible"
              n53 = call "Handle Error (User).vi"("error in"=w226, "Node in"=w227) -> ("error out"=w225:errorcluster, "Node out"=w224:refnum<class "BLS Chiller Template.lvclass">)  [unwired: 8 in]
              n54 = call <vilib>:"Log Error.vi"("Action"=Error_Options."Pause on Error", "error in (no error)"=w225, "Plug-in State in"=w220, "AdasLvTemplate in"=w223) -> ("error out"=w228:errorcluster, "Plug-in State out"=w222:T4, "AdasLvTemplate out"=w229:refnum<class "AdasLvTemplate.lvclass">)  [unwired: 5 in]
            }
          }
        }
      }
    }
    n55 = call "Cleanup (User).vi"("error in"=w37, "Node in"=w42) -> ("error in"=w47:errorcluster, "Node out"=w46:refnum<class "BLS Chiller Template.lvclass">)  [unwired: 8 in]
    n56 = Or(x=w34, y=w35) -> (x .or. y?=w45:bool)
    n57 = call "Specific Error Handler2"("Error to Check"=w34) -> ()  [unwired: 11 in, 4 out]
  }
  n58 = call "Register gRPC Events.vi"("error in"=w9, "Node in"=w7) -> ("error out"=w10:errorcluster, "Event Registration Refnum"=w18:refnum<event-registration>, "Node out"=w11:refnum<class "BLS Chiller Template.lvclass">)  [unwired: 7 in]
  n59 = case shown="No Error" w10 {
    selector: w10 -> [w298 w312]
    tunnel: w18 -> [w299 w313]
    tunnel: [w300 w313] -> w17
    tunnel: w11 -> [w301 _]
    tunnel: [w298 w312] -> w16
    frame No Error {
      n60 = while {
        tunnel: w299 -> [w308]
        shift-right: [w310] -> _
        shift-left: w301 -> [w306]
        tunnel: [w309] -> w300
        stop <- w307 stop-if-true
        # "Check for gRPC Server Events"
        # "OOB Comm to Main Loop"
        # "Transfer data to Main Loop if data updates."
        # "Custom gRPC Loop"
        n61 = local read "Main to gRPC"() -> (w305:T1)
        n62 = call "gRPC Data Transfer.vi"("Main to gRPC"=w305, "Node in"=w306) -> ("Update"=w302:bool, "Node out"=w304:refnum<class "BLS Chiller Template.lvclass">, "gRPC to Main"=w303:T2)  [unwired: 7 in]
        n63 = case shown="True" w302 {
          tunnel: w303 -> [_ w311]
          frame False {
          }
          frame True {
            n64 = local write "gRPC to Main"(w311) -> ()
          }
        }
        n65 = call "Custom gRPC Service Core.vi"("Event Registration Refnum in"=w308, "Node In"=w304) -> ("Server Stop"=w307:bool, "Node out"=w310:refnum<class "BLS Chiller Template.lvclass">, "Event Registration Refnum out"=w309:refnum<event-registration>)  [unwired: 7 in]
      }
    }
    frame Error {
    }
  }
  n66 = Unregister For Events(event registration refnum=w17, error in=w16) -> (error out=w15:errorcluster)
  n67 = call <vilib>:"Write AdasLvTemplate.vi"("error in"=w25, "AdasLvTemplate.lvlib:AdasLvTemplate.lvclass"=w27, "Template Node in"=w26) -> ("error out"=w2:errorcluster, "Template Node out"=w13:refnum<class "BLS Chiller Template.lvclass">)  [unwired: 7 in]
  n68 = call <vilib>:"Destroy Custom gRPC Service.vi"("Template Node in"=w13) -> ("error out"=w1:errorcluster, "Template Node out"=→"Node out":refnum<class "BLS Chiller Template.lvclass">)  [unwired: 9 in]
  n69 = Merge Errors(w2, w1, w15) -> (w14:errorcluster)
  n70 = call "Specific Error Handler"("Error to Check"=w14) -> ("error out"=→"error out":errorcluster)  [unwired: 11 in, 3 out]
